vi "CleanupString.vi"(1 "String":string) -> (0 "url":string)   [LabVIEW 2012]
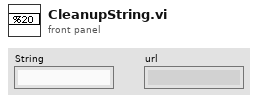
[diagram p1: front panel]
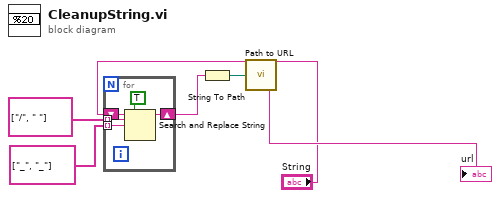
[diagram p0: block diagram]
diagram:
  n1 = for {
    tunnel: string[] ["/", " "] -> [w10] mode=indexing
    tunnel: string[] ["_", "_"] -> [w9] mode=indexing
    shift-right: [w7] -> w4
    shift-left: "String" -> [w8]
    n2 = Search and Replace String(replace all?=TRUE ("replace all? (F)"), input string=w8, search string=w10, replace string=w9) -> (result string=w7:string)  [unwired: 4 in, 3 out]
  }
  n3 = String To Path(string=w4) -> (path=w3:path)
  n4 = call <vilib>:"Path to URL.vi"("path"=w3) -> ("url"=→"url":string)
